vi "write_table_mode_command.vi"(10 "Synth Controls":T1={"Channel Settings"=[{"Voltage (Amp.) "=0.0, "Frequency (MHz)"=0.0, "Phase (deg)"=0.0, "Nickname"="Channel 0 D"}, {"Voltage (Amp.) "=0.0, "Frequency (MHz)"=0.0, "Phase (deg)"=0.0, "Nickname"="Channel 0 D"}, {"Voltage (Amp.) "=0.0, "Frequency (MHz)"=0.0, "Phase (deg)"=0.0, "Nickname"="Channel 0 D"}, {"Voltage (Amp.) "=0.0, "Frequency (MHz)"=0.0, "Phase (deg)"=0.0, "Nickname"="Channel 0 D"}], "Active Channels"=[TRUE, FALSE, FALSE, FALSE], "COM Port"="COM5", "Table Mode"={"Table Mode On/Off"=FALSE, "Initial Frequency (MHz)"=0.0, "FinalFreq"=0.0, "Frequency Step (MHz)"=0.0, "Ascending/Descending"=FALSE, "Random"=FALSE}}) -> (2 "Table Mode Command":string)   [LabVIEW 2015]
uses:
  Controls/Synth_409b/Synth_controls.ctl
  Controls/Synth_409b/synth_channel.ctl
  Controls/Synth_409b/table_mode.ctl
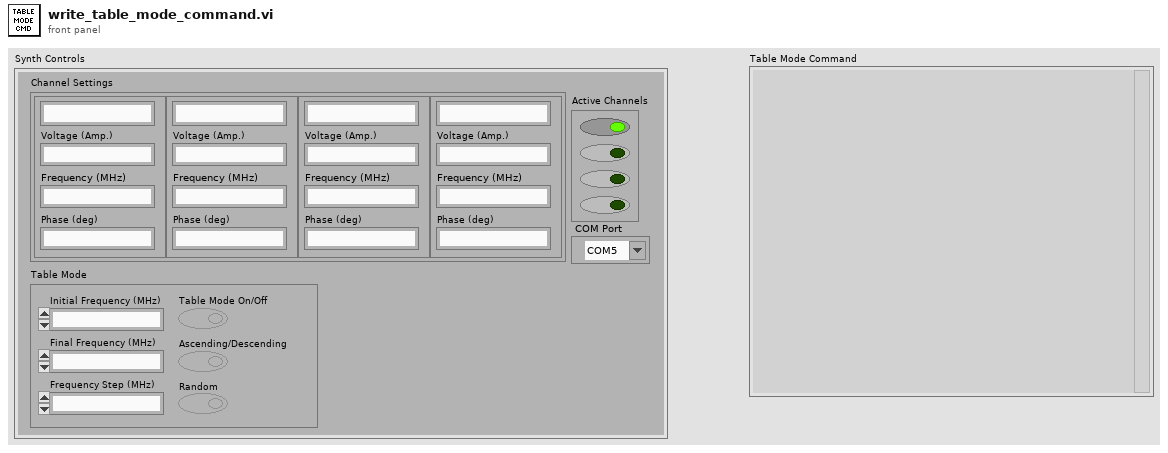
[diagram p1: front panel]
types:
  T1 = typedef "Synth_controls.ctl" = cluster{"Channel Settings":T2[], "Active Channels":bool[], "COM Port":refnum<visa-resource-name>, "Table Mode":T3}
  T2 = typedef "synth_channel.ctl" = cluster{"Voltage (Amp.) ":dbl, "Frequency (MHz)":dbl, "Phase (deg)":dbl, "Nickname":string}
  T3 = typedef "table_mode.ctl" = cluster{"Table Mode On/Off":bool, "Initial Frequency (MHz)":dbl, "FinalFreq":dbl, "Frequency Step (MHz)":dbl, "Ascending/Descending":bool, "Random":bool}
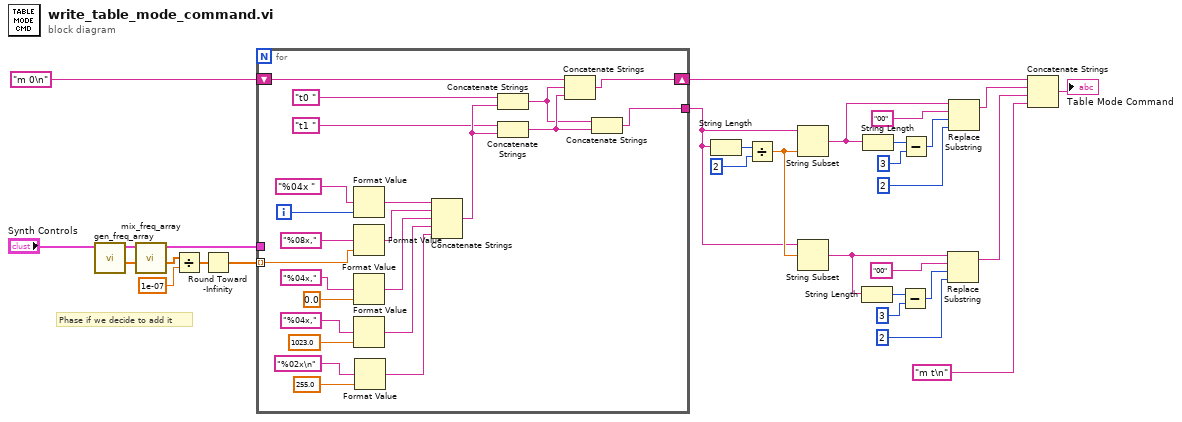
[diagram p0: block diagram]
diagram:
  # "Phase if we decide to add it"
  n1 = call "gen_freq_array.vi"("Synth Controls"="Synth Controls") -> ("Synth Controls Out"=w28:T1, "Array"=w29:dbl[])  [unwired: 8 in]
  n2 = call "mix_freq_array.vi"("Freq Array In"=w29, "Synth Controls"=w28) -> ("Mixed Freq Array"=w25:dbl[], "Synth Controls Out"=w26:T1)  [unwired: 8 in]
  n3 = Divide(x=w25, y=1e-07) -> (x/y=w23:dbl[])
  n4 = Round Toward -Infinity(1:w23) -> (0:w22:dbl[])
  n5 = for {
    shift-right: [w38] -> w16
    shift-left: "m 0\n" -> [w37]
    tunnel: w26 -> [_]
    tunnel: w22 -> [w50] mode=indexing
    tunnel: [w31] -> w3
    i -> [w53]
    n6 = Format Value(format string="%04x ", value (0)=w53) -> (output string=w51:string)  [unwired: 1 in]
    n7 = Format Value(format string="%08x,", value (0)=w50) -> (output string=w48:string)  [unwired: 1 in]
    n8 = Format Value(format string="%04x,", value (0)=0.0) -> (output string=w45:string)  [unwired: 1 in]
    n9 = Format Value(format string="%04x,", value (0)=1023.0) -> (output string=w42:string)  [unwired: 1 in]
    n10 = Format Value(format string="%02x\n", value (0)=255.0) -> (output string=w39:string)  [unwired: 1 in]
    n11 = Concatenate Strings(w51, w48, w45, w42, w39) -> (w36:string)
    n12 = Concatenate Strings("t0 ", w36) -> (w32:string)
    n13 = Concatenate Strings("t1 ", w36) -> (w33:string)
    n14 = Concatenate Strings(w37, w32, w33) -> (w38:string)
    n15 = Concatenate Strings(w32, w33) -> (w31:string)
  }
  n16 = String Length(string=w3) -> (length=w14:i32)
  n17 = Divide(x=w14, y=2) -> (x/y=w4:dbl)
  n18 = String Subset(string=w3, length (rest)=w4) -> (substring=w7:string)  [unwired: 1 in]
  n19 = String Subset(string=w3, offset (0)=w4) -> (substring=w2:string)  [unwired: 1 in]
  n20 = String Length(string=w2) -> (length=w20:i32)
  n21 = String Length(string=w7) -> (length=w11:i32)
  n22 = Subtract(x=w20, y=3) -> (x-y=w18:i32)
  n23 = Subtract(x=w11, y=3) -> (x-y=w9:i32)
  n24 = Replace Substring(2:2 ("length (len. of substring)"), 3:w18, 4:"00", 5:w2) -> (1:w6:string)  [unwired: 1 out]
  n25 = Replace Substring(2:2 ("length (len. of substring)"), 3:w9, 4:"00", 5:w7) -> (1:w5:string)  [unwired: 1 out]
  n26 = Concatenate Strings(w16, w5, w6, "m t\n") -> (→"Table Mode Command":string)
